vi "IND560 Serial Initialize.vi"(8 "Error In":errorcluster, 11 "VISA Refnum in":refnum<visa-resource-name>) -> (0 "Error Out":errorcluster, 3 "VISA Refnum Out":refnum<visa-resource-name>)   [LabVIEW 2016]
uses:
  <vilib>/Instr/_visa.llb/VISA Configure Serial Port (Instr).vi
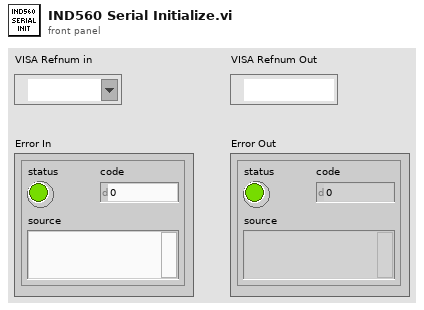
[diagram p1: front panel]
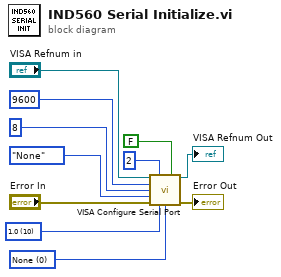
[diagram p0: block diagram]
diagram:
  w4 = u16 0 items=["None", "XON/XOFF", "RTS/CTS", "XON/XOFF & RTS/CTS", "DTR/DSR", "XON/XOFF & DTR/DSR"] ("flow control (0:none)")
  w5 = u16 10 items=["1.0"=10, "1.5"=15, "2.0"=20] ("stop bits (10: 1 bit)")
  n1 = call-poly "VISA Configure Serial Port"("VISA resource name"="VISA Refnum in", "timeout (10sec)"=u32 2, "Enable Termination\nChar (T)"=FALSE ("Enable Termination\nChar (T)"), "baud rate (9600)"=u32 9600, "data bits (8)"=u16 8, "parity (0:none)"=enum16{"None", "Odd", "Even", "Mark", "Space"}."None", "error in (no error)"="Error In", "stop bits (10: 1 bit)"=w5, "flow control (0:none)"=w4) -> ("VISA resource name out"=→"VISA Refnum Out":refnum<visa-resource-name>, "error out"=→"Error Out":errorcluster)  [unwired: 5 in]
